vi "WriteLinescanHeader.vi"(1 "error in":errorcluster, 2 "Destination:":path, 3 "Image Settings":T2={"Start Position (µm)"={"x"=0.0, "y"=0.0, "z"=0.0}, "End Position (µm)"={"x"=10.0, "y"=10.0, "z"=0.0}, "Image Resolution (nm/pixel)"={"x"=50.0, "y"=50.0, "z"=100.0}, "Image Size (µm)"={"x"=10.0, "y"=10.0, "z"=0.0}, "Image Size (pixel)"={"x"=50, "y"=50, "z"=0}, "Time Resolution\n(ms/pixel)"=7.0, "1st Axis"=0, "2nd Axis"=1, "Retrace"=FALSE, "Estimated Time"=""} {"2nd Axis" items=["x", "y", "z"]; "1st Axis" items=["x", "y", "z"]; "Time Resolution\n(ms/pixel)" format="%.2f"; "Image Resolution (nm/pixel)"."z" format="%.2f"; "Image Resolution (nm/pixel)"."y" format="%.2f"; "Image Resolution (nm/pixel)"."x" format="%.2f"; "Image Size (µm)"."z" format="%.2f"; "Image Size (µm)"."y" format="%.2f"; "Image Size (µm)"."x" format="%.2f"; "End Position (µm)"."z" format="%.2f"; "End Position (µm)"."y" format="%.2f"; "End Position (µm)"."x" format="%.2f"; "Start Position (µm)"."z" format="%.2f"; "Start Position (µm)"."y" format="%.2f"; "Start Position (µm)"."x" format="%.2f"}) -> (0 "error out":errorcluster)   [LabVIEW 2009]
uses:
  FIFOSettings.ctt
  ImageSettings.ctt
  FIFOSettings_SPC.ctt
  <vilib>/Utility/xml.llb/Write to XML File(string).vi
panel:
  in  "FIFO Settings SPC":T1={"Measurement"={"Binning (ms)"=0.001, "External Trigger Condition"=0, "Stop Condition:"=0, "Stop Count"=0.0, "Buffer Size (Photons)"=30000, "No of Channels"=1, "Ext Latch Delay"=0}, "ADC"={"Module"=0, "ADC Resolution"=1, "Dither Range"=0, "Count Increment"=1, "Macro Time Clock"=0}, "SYNC"={"SYNC ZC Level (mV)"=-49.889763, "SYNC Freq Divider"=1, "SYNC Holdoff (ns)"=4.0, "SYNC Threshold (mV)"=-19.607843}, "TAC"={"TAC Range (ns)"=50.0, "TAC Gain"=1, "TAC Offset (%)"=0.0, "TAC Limit Low (%)"=0.0, "TAC Limit High (%)"=100.0}, "CFD"={"CFD Limit Low (mV)"=-43.137257, "CFD Limit High (mV)"=67.76471, "CFD ZC Level (mV)"=-49.889763, "CFD Holdoff (ns)"=5.0}} {"CFD"."CFD Holdoff (ns)" min=5 max=20 format="%.2f"; "CFD"."CFD ZC Level (mV)" min=-96 max=96 format="%.2f"; "CFD"."CFD Limit High (mV)" min=4 max=80 format="%.2f"; "CFD"."CFD Limit Low (mV)" min=-500 max=80 format="%.2f"; "TAC"."TAC Limit High (%)" min=0 max=100 format="%.2f"; "TAC"."TAC Limit Low (%)" min=0 max=100 format="%.2f"; "TAC"."TAC Offset (%)" min=0 max=100 format="%.2f"; "TAC"."TAC Gain" min=1 max=15 step=1; "TAC"."TAC Range (ns)" min=50 max=2000 format="%.2f"; "SYNC"."SYNC Threshold (mV)" min=-500 max=-19 format="%.2f"; "SYNC"."SYNC Holdoff (ns)" min=4 max=16 format="%.2f"; "SYNC"."SYNC Freq Divider" min=1 max=16 step=1; "SYNC"."SYNC ZC Level (mV)" min=-96 max=96 format="%.2f"; "ADC"."Macro Time Clock" items=["Internal (50ns)", "Sync-Trigger", "1/2 Sync-Trigger"]; "ADC"."Module" items=["SPC 630", "SPC 830", "SPC 13x", "HydraHarp"]; "ADC"."Count Increment" min=1 max=255 step=1; "ADC"."Dither Range" min=0 max=256 step=32; "Measurement"."Ext Latch Delay" min=0 max=255 step=1; "Measurement"."Stop Count" format="%.2f"; "Measurement"."Stop Condition:" items=["None", "Photon Count", "Time (s)"]; "Measurement"."External Trigger Condition" max=2 step=1; "Measurement"."No of Channels" max=14; "Measurement"."Binning (ms)" min=1e-07 max=100000 format="%.3f"}
  out "FIFO Settings HH":T3={"Measurement"={"Binning (ms)"=0.001, "External Trigger Condition"=0, "Stop Condition:"=0, "Stop Count"=0.0, "Buffer Size (Photons)"=30000, "No of Channels"=1, "Ext Latch Delay"=0}, "ADC"={"Binning (HH)"=12, "Dither Range"=0, "Count Increment"=1, "Mode"=1}, "SYNC"={"SYNC ZC Level (mV)"=-49.889763, "SYNC Freq Divider"=1, "SYNC Holdoff (ps)"=4.0, "SYNC Threshold (mV)"=-19.607843}, "TAC"={"TAC Range (ns)"=50.0, "TAC Gain"=2, "TAC Offset (%)"=0.0, "TAC Limit Low (%)"=0.0, "TAC Limit High (%)"=100.0}, "Ch 2"={"Ch2 ZC Level (mV)"=-43.137257, "Ch2 Holdoff (ps)"=67.76471, "Ch2 Threshold (mV)"=-49.889763}, "Ch 3"={"Ch3 ZC Level (mV)"=10.0, "Ch3 Holdoff (ps)"=0.0, "Ch3 Threshold (mV)"=200.0}, "Ch 4"={"Ch4 ZC Level (mV)"=10.0, "Ch4 Holdoff (ps)"=0.0, "Ch4 Threshold (mV)"=200.0}, "Ch1"={"Ch1 ZC Level (mV)"=10.0, "Ch1 Holdoff (ps)"=0.0, "Ch1 Threshold (mV)"=200.0}} {"Ch1"."Ch1 Threshold (mV)" min=0 max=1000 format="%.2f"; "Ch1"."Ch1 Holdoff (ps)" min=-99999 max=99999 format="%.2f"; "Ch1"."Ch1 ZC Level (mV)" min=0 max=40 format="%.2f"; "Ch 4"."Ch4 Threshold (mV)" min=0 max=1000 format="%.2f"; "Ch 4"."Ch4 Holdoff (ps)" min=-99999 max=99999 format="%.2f"; "Ch 4"."Ch4 ZC Level (mV)" min=0 max=40 format="%.2f"; "Ch 3"."Ch3 Threshold (mV)" min=0 max=1000 format="%.2f"; "Ch 3"."Ch3 Holdoff (ps)" min=-99999 max=99999 format="%.2f"; "Ch 3"."Ch3 ZC Level (mV)" min=0 max=40 format="%.2f"; "Ch 2"."Ch2 Threshold (mV)" min=-96 max=96 format="%.2f"; "Ch 2"."Ch2 Holdoff (ps)" min=4 max=80 format="%.2f"; "Ch 2"."Ch2 ZC Level (mV)" min=-500 max=80 format="%.2f"; "TAC"."TAC Limit High (%)" min=0 max=100 format="%.2f"; "TAC"."TAC Limit Low (%)" min=0 max=100 format="%.2f"; "TAC"."TAC Offset (%)" min=0 max=100 format="%.2f"; "TAC"."TAC Gain" min=1 max=15 step=1; "TAC"."TAC Range (ns)" min=50 max=2000 format="%.2f"; "SYNC"."SYNC Threshold (mV)" min=-500 max=-19 format="%.2f"; "SYNC"."SYNC Holdoff (ps)" min=4 max=16 format="%.2f"; "SYNC"."SYNC Freq Divider" items=["1", "2", "4", "8", "16"]; "SYNC"."SYNC ZC Level (mV)" min=-96 max=96 format="%.2f"; "ADC"."Mode" items=["T3"]; "ADC"."Binning (HH)" items=["1", "2", "4", "8", "16", "32", "64", "128", "256", "512", "1024"]; "ADC"."Count Increment" min=1 max=255 step=1; "ADC"."Dither Range" min=0 max=256 step=32; "Measurement"."Ext Latch Delay" min=0 max=255 step=1; "Measurement"."Stop Count" format="%.2f"; "Measurement"."Stop Condition:" items=["None", "Photon Count", "Time (s)"]; "Measurement"."External Trigger Condition" max=2 step=1; "Measurement"."No of Channels" max=14; "Measurement"."Binning (ms)" min=1e-07 max=100000 format="%.3f"}
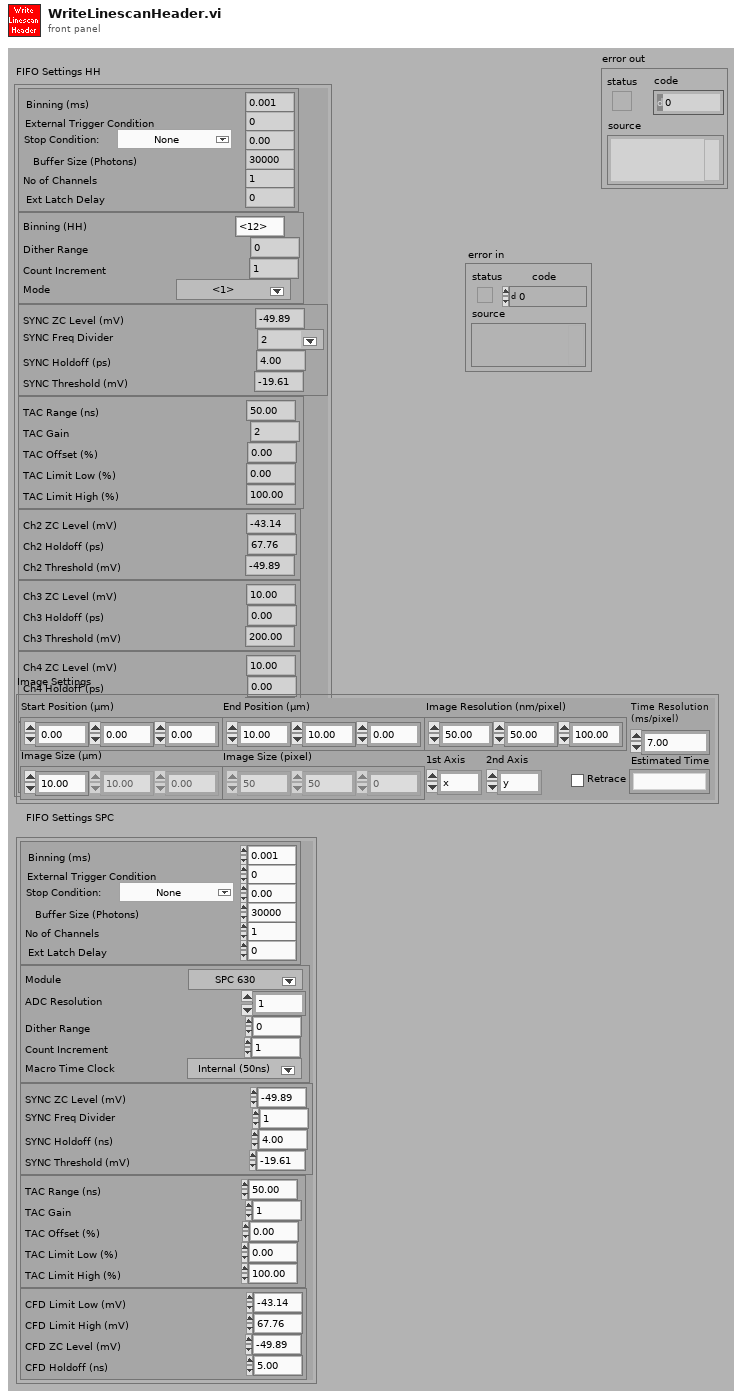
[diagram p1: front panel]
types:
  T1 = typedef "FIFOSettings_SPC.ctt" = cluster{"Measurement":cluster{"Binning (ms)":sgl, "External Trigger Condition":u16, "Stop Condition:":u16, "Stop Count":dbl, "Buffer Size (Photons)":u16, "No of Channels":u16, "Ext Latch Delay":i16}, "ADC":cluster{"Module":u16, "ADC Resolution":i32, "Dither Range":i16, "Count Increment":i16, "Macro Time Clock":i16}, "SYNC":cluster{"SYNC ZC Level (mV)":sgl, "SYNC Freq Divider":i16, "SYNC Holdoff (ns)":sgl, "SYNC Threshold (mV)":sgl}, "TAC":cluster{"TAC Range (ns)":sgl, "TAC Gain":i16, "TAC Offset (%)":sgl, "TAC Limit Low (%)":sgl, "TAC Limit High (%)":sgl}, "CFD":cluster{"CFD Limit Low (mV)":sgl, "CFD Limit High (mV)":sgl, "CFD ZC Level (mV)":sgl, "CFD Holdoff (ns)":sgl}}
  T2 = typedef "ImageSettings.ctt" = cluster{"Start Position (µm)":cluster{"x":dbl, "y":dbl, "z":dbl}, "End Position (µm)":cluster{"x":dbl, "y":dbl, "z":dbl}, "Image Resolution (nm/pixel)":cluster{"x":dbl, "y":dbl, "z":dbl}, "Image Size (µm)":cluster{"x":dbl, "y":dbl, "z":dbl}, "Image Size (pixel)":cluster{"x":u32, "y":u32, "z":u32}, "Time Resolution\n(ms/pixel)":dbl, "1st Axis":u16, "2nd Axis":u16, "Retrace":bool, "Estimated Time":string}
  T3 = typedef "FIFOSettings.ctt" = cluster{"Measurement":cluster{"Binning (ms)":sgl, "External Trigger Condition":u16, "Stop Condition:":u16, "Stop Count":dbl, "Buffer Size (Photons)":u32, "No of Channels":u16, "Ext Latch Delay":i16}, "ADC":cluster{"Binning (HH)":i16, "Dither Range":i16, "Count Increment":i16, "Mode":u16}, "SYNC":cluster{"SYNC ZC Level (mV)":sgl, "SYNC Freq Divider":u16, "SYNC Holdoff (ps)":sgl, "SYNC Threshold (mV)":sgl}, "TAC":cluster{"TAC Range (ns)":sgl, "TAC Gain":i16, "TAC Offset (%)":sgl, "TAC Limit Low (%)":sgl, "TAC Limit High (%)":sgl}, "Ch 2":cluster{"Ch2 ZC Level (mV)":sgl, "Ch2 Holdoff (ps)":sgl, "Ch2 Threshold (mV)":sgl}, "Ch 3":cluster{"Ch3 ZC Level (mV)":sgl, "Ch3 Holdoff (ps)":sgl, "Ch3 Threshold (mV)":sgl}, "Ch 4":cluster{"Ch4 ZC Level (mV)":sgl, "Ch4 Holdoff (ps)":sgl, "Ch4 Threshold (mV)":sgl}, "Ch1":cluster{"Ch1 ZC Level (mV)":sgl, "Ch1 Holdoff (ps)":sgl, "Ch1 Threshold (mV)":sgl}}
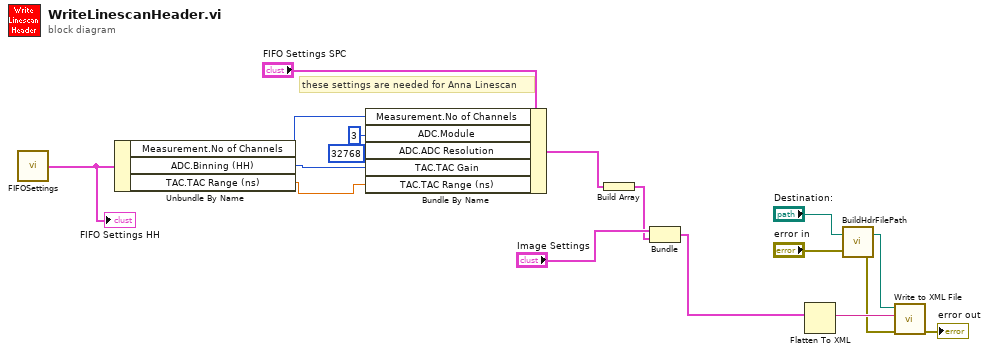
[diagram p0: block diagram]
diagram:
  # "these settings are needed for Anna Linescan"
  n1 = call "FIFOSettings.vi"() -> ("FIFO Settings(out)"=w10:T3)  [unwired: 2 in]
  "FIFO Settings HH" <- w10
  n2 = Unbundle By Name(w10) -> ("Measurement.No of Channels"=w4:u16, "ADC.Binning (HH)"=w1:i16, "TAC.TAC Range (ns)"=w5:sgl)
  n3 = Bundle By Name(cluster="FIFO Settings SPC", "Measurement.No of Channels"=w4, "ADC.Module"=u16 3, "ADC.ADC Resolution"=32768, "TAC.TAC Gain"=w1, "TAC.TAC Range (ns)"=w5) -> (w6:T1)
  n4 = Build Array(w6) -> (w8:T1[])
  n5 = Bundle("Image Settings"="Image Settings", w8) -> (w7:cluster{"Image Settings":T2, T1[]})  [unwired: 1 in]
  n6 = Flatten To XML(anything=w7) -> (xml string=w15:string)
  n7 = call "BuildHdrFilePath.vi"("error in"="error in", "Destination:"="Destination:") -> ("error in (no error)"=w3:errorcluster, "configuration file path"=w14:path)
  n8 = call-poly <vilib>:"Write to XML File.vi"("error in (no error)"=w3, "XML Input"=w15, "XML File Path"=w14) -> ("error out"=→"error out":errorcluster)  [unwired: 6 in, 2 out]
